vi "Init.vi"(8 "error in (no error)":errorcluster, 10 "Channel":i16=-10, 11 "AODAcq in":refnum<class "AODAcq.lvclass">) -> (0 "error out":errorcluster, 3 "AODAcq out":refnum<class "AODAcq.lvclass">)   [LabVIEW 2014, in "AODAcq.lvclass"]
uses:
  AODAcq.lvclass
  AcquistionObject/AcquistionObject.lvclass
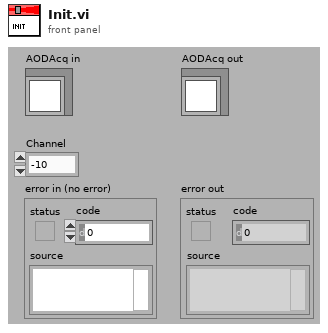
[diagram p1: front panel]
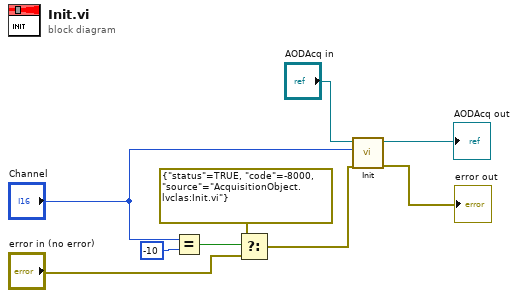
[diagram p0: block diagram]
diagram:
  n1 = Equal?(x="Channel", y=i16 -10 ("x")) -> (x = y?=w8:bool)
  n2 = Select(t=errorcluster {"status"=TRUE, "code"=-8000, "source"="AcquisitionObject.lvclas:Init.vi"}, s=w8, f="error in (no error)") -> (s? t:f=w3:errorcluster)
  n3 = call-parent "Init.vi"("error in (no error)"=w3, "Channel"="Channel", "AcquistionObject in"="AODAcq in") -> ("error out"=→"error out":errorcluster, "AcquistionObject out"=→"AODAcq out":refnum<class "AODAcq.lvclass">)  [unwired: 7 in]
